vi "Terminate.vi"(8 "error in (no error)":errorcluster, 10 "Message in":refnum<class "TerminateMessage.lvclass">, 11 "DAQCascade512II in":refnum<class "DAQCascade512II.lvclass">) -> (0 "error out":errorcluster, 3 "DAQCascade512II out":refnum<class "DAQCascade512II.lvclass">)   [LabVIEW 2012, in "DAQCascade512II.lvclass"]
doc: "This member function is called when the statemachine in the run.vi receives an 'terminate' command. It closes the RabbitMQ connection. \n\nOverride this member function in your derived class to release all previously acquired resources (but don't forget to call the parent method). If your component has subcomponents, they count as resources, and you have to release them by calling their own terminate functions."
uses:
  DAQCascade512II.lvclass
  <vilib>/Distrio/Murmex/TerminateMessage/TerminateMessage.lvclass
  run_time cluster.ctl
  <vilib>/vision/Image Controls.llb/IMAQ Image.ctl
  DAQCascade512II.lvclass/DAQCascade512II.ctl
  <vilib>/Distrio/Murmex/Murmex/Murmex.lvclass
panel:
  in  "run time":T1
  in  "error in":errorcluster
  # "This method is called when the TERMINATE\ntrigger is sent. \n\nOverride this method when your component needs to\nrespond to this trigger. \n\nCall parent for proper implementation"
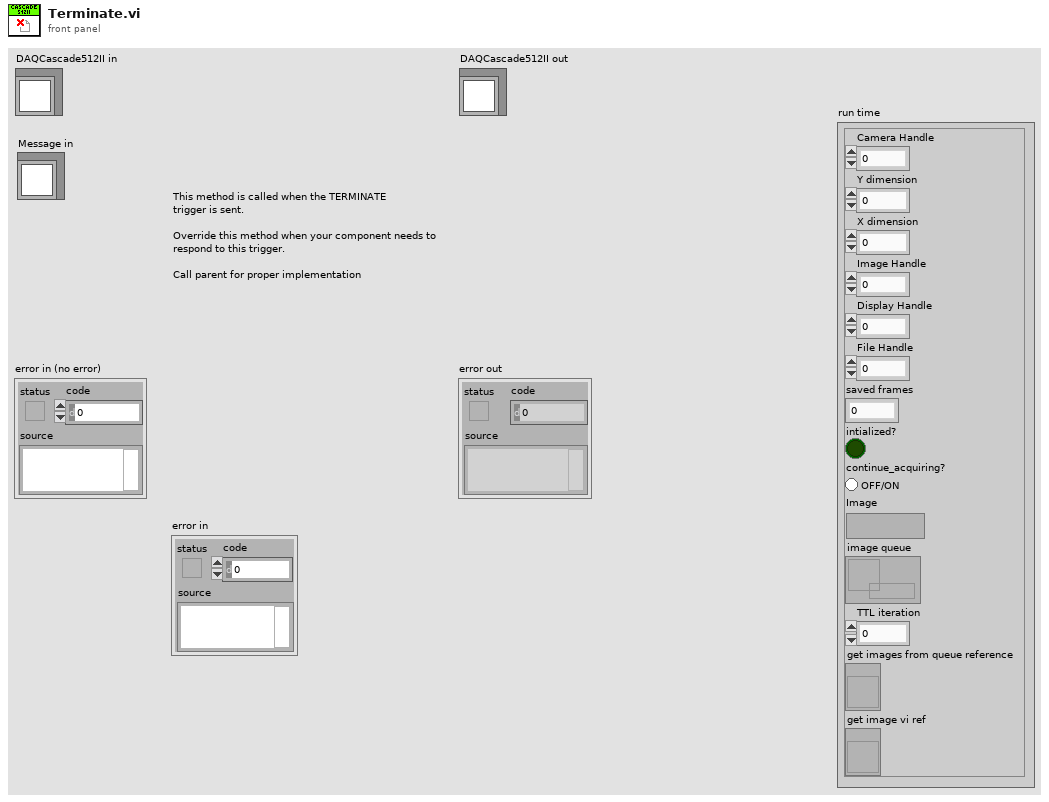
[diagram p1: front panel]
types:
  T1 = typedef "DAQCascade512II.lvclass/run_time cluster.ctl" = cluster{"Camera Handle":u32, "Y dimension":u32, "X dimension":u32, "Image Handle":u32, "Display Handle":u32, "File Handle":u32, "saved frames":dbl, "intialized?":bool, "continue_acquiring?":bool, "Image":T2, "image queue":refnum<queue>, "TTL iteration":i32, "get images from queue reference":refnum<vi>, "get image vi ref":refnum<vi>}
  T2 = typedef "IMAQ Image.ctl" = refnum<image>
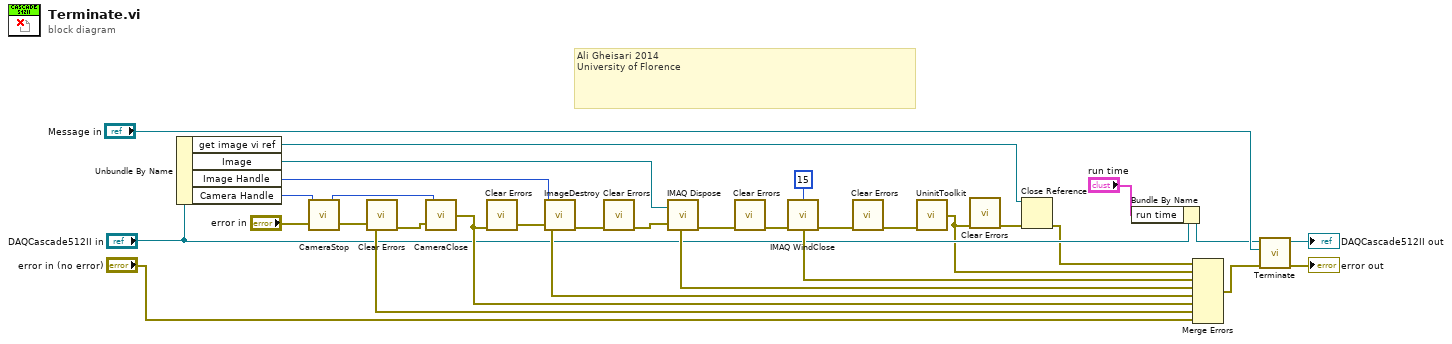
[diagram p0: block diagram]
diagram:
  # "Ali Gheisari 2014\nUniversity of Florence"
  n1 = Unbundle By Name("DAQCascade512II in") -> ("get image vi ref"=w4:refnum<vi>, "Image"=w11:T2, "Image Handle"=w24:u32, "Camera Handle"=w18:u32)
  n2 = call <userlib>:"CameraStop.vi"("error in"="error in", "Camera Handle"=w18) -> ("error out"=w19:errorcluster, "Camera Handle"=w25:u32)
  n3 = call <vilib>:"Clear Errors.vi"("error in (no error)"=w19) -> ("error out"=w26:errorcluster)  [unwired: 6 in]
  n4 = call <userlib>:"CameraClose.vi"("error in"=w26, "Camera Handle"=w25) -> ("error out"=w20:errorcluster)
  n5 = call <vilib>:"Clear Errors.vi"("error in (no error)"=w20) -> ("error out"=w15:errorcluster)  [unwired: 6 in]
  n6 = call <userlib>:"ImageDestroy.vi"("error in"=w15, "Data handle"=w24) -> ("error out"=w21:errorcluster)
  n7 = call <vilib>:"Clear Errors.vi"("error in (no error)"=w21) -> ("error out"=w13:errorcluster)  [unwired: 6 in]
  n8 = call "IMAQ Dispose"("Image"=w11, "error in (no error)"=w13) -> ("error out"=w12:errorcluster)  [unwired: 4 in]
  n9 = call <vilib>:"Clear Errors.vi"("error in (no error)"=w12) -> ("error out"=w14:errorcluster)  [unwired: 6 in]
  n10 = call "IMAQ WindClose"("Window Number (0...15)"=15, "error in (no error)"=w14) -> ("error out"=w9:errorcluster)  [unwired: 4 in]
  n11 = call <vilib>:"Clear Errors.vi"("error in (no error)"=w9) -> ("error out"=w10:errorcluster)  [unwired: 6 in]
  n12 = call <userlib>:"UninitToolkit.vi"("error in"=w10) -> ("error out"=w3:errorcluster)
  n13 = call <vilib>:"Clear Errors.vi"("error in (no error)"=w3) -> ("error out"=w2:errorcluster)  [unwired: 6 in]
  n14 = Close Reference(reference=w4, error in (no error)=w2) -> (error out=w1:errorcluster)
  n15 = Bundle By Name(cluster="DAQCascade512II in", "run time"="run time") -> (w6:refnum<class "DAQCascade512II.lvclass">)
  n16 = Merge Errors(w1, w3, w9, w12, w21, w20, w19, "error in (no error)") -> (w17:errorcluster)
  n17 = call-parent "Terminate.vi"("error in (no error)"=w17, "Message in"="Message in", "Murmex in"=w6) -> ("error out"=→"error out":errorcluster, "Murmex out"=→"DAQCascade512II out":refnum<class "DAQCascade512II.lvclass">)  [unwired: 7 in]
